vi "WPI_JoystickButtonSpinMapping.vi"(6 "Max Output":dbl=1.0, 7 "Square Inputs":bool=TRUE, 8 "Spin?":bool, 9 "Y axis value":dbl, 10 "X axis value":dbl) -> (2 "Right Motor Value":dbl, 3 "Left Motor Value":dbl)   [LabVIEW 2017]
doc: "A variation of the standard algorithm to map joystick axes into motor updates for arcade driving. This VI also allows you to control the spinning direction of motors on either side of the robot."
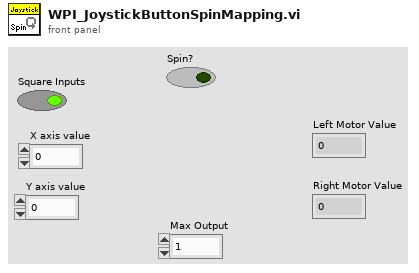
[diagram p1: front panel]
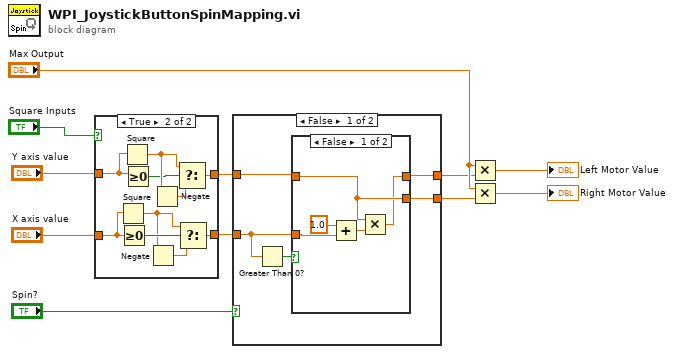
[diagram p0: block diagram]
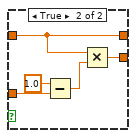
[diagram p3: hidden frame]
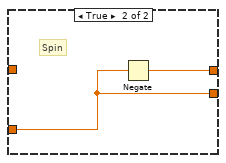
[diagram p4: hidden frame]
diagram:
  n1 = case shown="True" "Square Inputs" {
    tunnel: [w12 w23] -> w2
    tunnel: [w13 w22] -> w4
    tunnel: "X axis value" -> [w12 w21]
    tunnel: "Y axis value" -> [w13 w20]
    frame False {
    }
    frame True {
      n2 = Square(x=w21) -> (x^2=w18:dbl)
      n3 = Greater Or Equal To 0?(x=w21) -> (x >= 0?=w19:bool)
      n4 = Square(x=w20) -> (x^2=w15:dbl)
      n5 = Greater Or Equal To 0?(x=w20) -> (x >= 0?=w14:bool)
      n6 = Negate(x=w18) -> (-x=w17:dbl)
      n7 = Negate(x=w15) -> (-x=w16:dbl)
      n8 = Select(t=w15, s=w14, f=w16) -> (s? t:f=w22:dbl)
      n9 = Select(t=w18, s=w19, f=w17) -> (s? t:f=w23:dbl)
    }
  }
  n10 = case shown="False" "Spin?" {
    tunnel: w4 -> [w27 _]
    tunnel: [w26 w40] -> w3
    tunnel: w2 -> [w24 w39]
    tunnel: [w25 w39] -> w9
    frame False {
      n11 = Greater Than 0?(x=w24) -> (x > 0?=w28:bool)
      n12 = case shown="False" w28 {
        tunnel: w27 -> [w33 w38]
        tunnel: [w32 w38] -> w26
        tunnel: w24 -> [w31 w36]
        tunnel: [w33 w34] -> w25
        frame False {
          n13 = Add(x=1.0, y=w31) -> (x+y=w29:dbl)
          n14 = Multiply(x=w33, y=w29) -> (x*y=w32:dbl)
        }
        frame True {
          n15 = Subtract(x=1.0, y=w36) -> (x-y=w35:dbl)
          n16 = Multiply(x=w38, y=w35) -> (x*y=w34:dbl)
        }
      }
    }
    frame True {
      # "Spin"
      n17 = Negate(x=w39) -> (-x=w40:dbl)
    }
  }
  n18 = Multiply(x="Max Output", y=w3) -> (x*y=→"Left Motor Value":dbl)
  n19 = Multiply(x="Max Output", y=w9) -> (x*y=→"Right Motor Value":dbl)
